vi "zmq REQ dup.vi"() -> ()   [LabVIEW 2015]
uses:
  <vilib>/addons/zeromq/poll_type.ctl
  <vilib>/addons/zeromq/socket_type.ctl
  <vilib>/addons/zeromq/zmq_context.lvclass
  <vilib>/addons/zeromq/zeromq.lvlib
  <vilib>/addons/zeromq/zmq_socket.lvclass
panel:
  in  "Connection Type":enum16{"connect", "bind"}(ring)
  in  "Poll":bool
  out "timed out?":bool
  out "nevents":i32
  out "polled events":T1[](array[typedef])
  in  "poll type":T1=enum."In/Out"
  in  "receive":bool
  in  "Message":string="{\"msg_id\":\"555\",\"msg_type\":\"read\",\"msg_property\":\"vmon\",\"8-04\":\"XXX\"}"
  in  "SEND":bool
  out "HB":bool
  out "error out":errorcluster
  in  "stop":bool
  in  "ZMQ endpoint":string="tcp://127.0.0.1:5555"
  out "REPLY":string
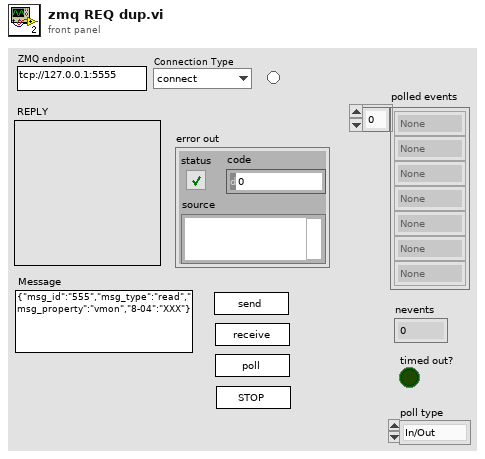
[diagram p1: front panel]
types:
  T1 = typedef "zeromq.lvlib/poll_type.ctl" = enum16{"None", "In", "Out", "In/Out"}
  T2 = typedef "zeromq.lvlib/socket_type.ctl" = enum8{"ZMQ_PAIR", "ZMQ_PUB", "ZMQ_SUB", "ZMQ_REQ", "ZMQ_REP", "ZMQ_DEALER", "ZMQ_ROUTER", "ZMQ_PULL", "ZMQ_PUSH", "ZMQ_XPUB", "ZMQ_XSUB"}
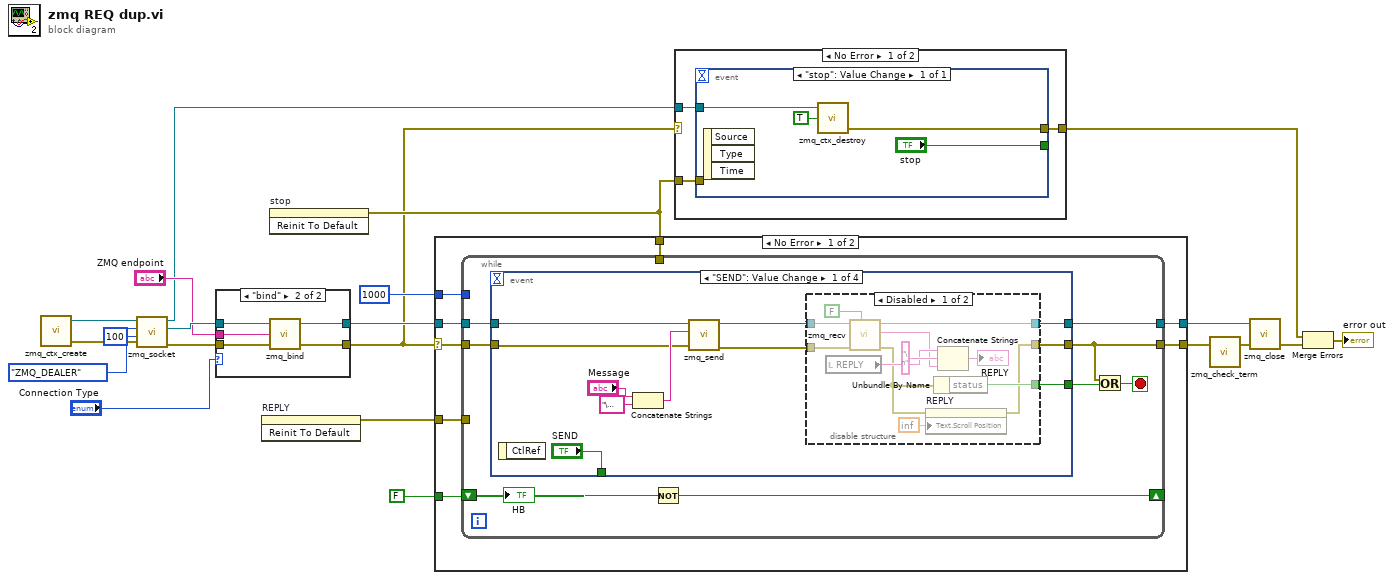
[diagram p0: block diagram]
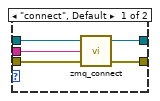
[diagram p2: hidden frame]
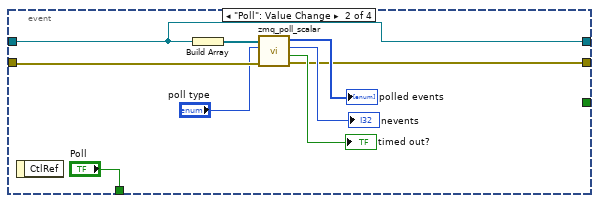
[diagram p4: hidden frame]
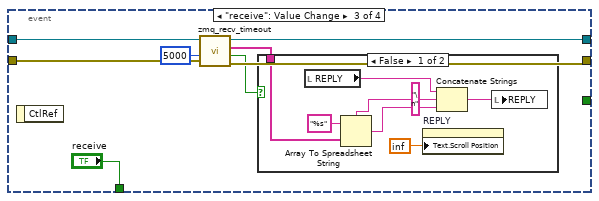
[diagram p5: hidden frame]
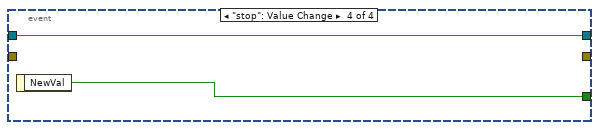
[diagram p7: hidden frame]
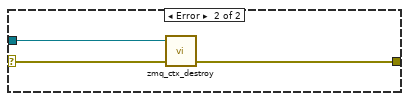
[diagram p9: hidden frame]
diagram:
  n1 = call <vilib>:"zmq_ctx_create.vi"() -> ("error out"=w14:errorcluster, "context out"=w12:refnum<class "zmq_context.lvclass">)  [unwired: 4 in]
  n2 = call <vilib>:"zmq_socket.vi"("error in"=w14, "linger (ms)"=100, "socket type"=socket_type."ZMQ_DEALER", "context in"=w12) -> ("error out"=w19:errorcluster, "socket out"=w20:refnum<class "zmq_socket.lvclass">, "context out"=w1:refnum<class "zmq_context.lvclass">)  [unwired: 1 in]
  n3 = case shown="\"bind\"" "Connection Type" {
    tunnel: w20 -> [w26 w31]
    tunnel: w19 -> [w25 w28]
    tunnel: [w24 w30] -> w18
    tunnel: "ZMQ endpoint" -> [w23 w27]
    tunnel: [w22 w29] -> w3
    frame "connect", Default {
      n4 = call <vilib>:"zmq_connect.vi"("error in"=w25, "endpoint"=w23, "socket in"=w26) -> ("error out"=w22:errorcluster, "socket out"=w24:refnum<class "zmq_socket.lvclass">)  [unwired: 1 in]
    }
    frame "bind" {
      n5 = call <vilib>:"zmq_bind.vi"("error in"=w28, "endpoint"=w27, "socket in"=w31) -> ("error out"=w29:errorcluster, "socket out"=w30:refnum<class "zmq_socket.lvclass">)  [unwired: 1 in]
    }
  }
  n6 = invoke on="REPLY" class="Str" method="Reinit To Default"() -> (error out=w13:errorcluster)  [unwired: 3 in, 2 out]
  n7 = invoke on="stop" class="Bool" method="Reinit To Default"() -> (error out=w5:errorcluster)  [unwired: 3 in, 2 out]
  n8 = case shown="No Error" w3 {
    selector: w3 -> [w32 w100]
    tunnel: w18 -> [w39 w99]
    tunnel: 1000 -> [w38 _]
    tunnel: [w37 w99] -> w16
    tunnel: w13 -> [w36 _]
    tunnel: [w35 w100] -> w11
    tunnel: FALSE ("stop") -> [w34 _]
    tunnel: w5 -> [w33 _]
    frame No Error {
      n9 = while {
        tunnel: w39 -> [w47]
        tunnel: w32 -> [w46]
        tunnel: w38 -> [_]
        tunnel: [w45] -> w37
        tunnel: [w40] -> w35
        tunnel: w36 -> [_]
        shift-right: [w43] -> _
        shift-left: w34 -> [w44]
        tunnel: w33 -> [_]
        stop <- w42 stop-if-true
        n10 = event shown="[0] \"SEND\": Value Change" {
          selector: _ -> [_ _ _ _]
          dyn-events: _ -> [_ _ _ _]
          timeout: _ -> [_ _ _ _]
          tunnel: [w57 _ _ w97] -> w41
          tunnel: w47 -> [w48 w75 w89 w98]
          tunnel: w46 -> [w49 w76 w88 _]
          tunnel: [w56 w75 w85 w98] -> w45
          tunnel: [w50 w74 w86 _] -> w40
          tunnel: ["SEND" "Poll" "receive" _] -> _
          event "SEND": Value Change {
            n11 = event-data() -> ()  [unwired: 1 in, 1 out]
            n12 = Concatenate Strings("Message", "\u0000" ("string")) -> (w51:string)
            n13 = call <vilib>:"zmq_send.vi"("error in"=w49, "data"=w51, "socket in"=w48) -> ("error out"=w55:errorcluster, "socket out"=w58:refnum<class "zmq_socket.lvclass">)  [unwired: 4 in]
            n14 = disable-structure shown="Disabled" {
              disable-tunnel: w58 -> [w70 w72]
              disable-tunnel: [w69 _] -> w57
              disable-tunnel: [w68 w72] -> w56
              disable-tunnel: w55 -> [w66 w71]
              disable-tunnel: [w59 w71] -> w50
              frame Disabled {
                n15 = local read "REPLY"() -> (w62:string)
                n16 = call <vilib>:"zmq_recv.vi"("no block? (F)"=FALSE, "error in"=w66, "socket in"=w70) -> ("error out"=w60:errorcluster, "data"=w61:string, "socket out"=w68:refnum<class "zmq_socket.lvclass">)  [unwired: 2 in, 2 out]
                n17 = property on="REPLY" class="Str"(error in=w60, "Text.Scroll Position"=inf) -> (error out=w59:errorcluster)  [unwired: 1 in, 1 out]
                n18 = Unbundle By Name(w60) -> ("status"=w69:bool)
                n19 = Concatenate Strings(w62, "\n" ("string"), w61) -> (→"REPLY":string)
              }
              frame Enabled {
              }
            }
          }
          event "Poll": Value Change {
            n20 = event-data() -> ()  [unwired: 1 in, 1 out]
            n21 = Build Array(w75) -> (w80:refnum<class "zmq_socket.lvclass">[])
            n22 = call <vilib>:"zmq_poll_scalar.vi"("error in"=w76, "poll type"="poll type", "sockets"=w80) -> ("error out"=w74:errorcluster, "timed out?"=→"timed out?":bool, "nevents"=→"nevents":i32, "polled events"=→"polled events":T1[])  [unwired: 1 in]
          }
          event "receive": Value Change {
            n23 = event-data() -> ()  [unwired: 1 in, 1 out]
            n24 = call <vilib>:"zmq_recv_timeout.vi"("error in"=w88, "timeout (ms)"=u32 5000, "socket in"=w89) -> ("error out"=w86:errorcluster, "timeout?"=w83:bool, "parts"=w84:string[], "socket out"=w85:refnum<class "zmq_socket.lvclass">)  [unwired: 1 in]
            n25 = case shown="False" w83 {
              tunnel: w84 -> [w92 _]
              frame False {
                w93 = "\n" ("string")
                n26 = local read "REPLY"() -> (w95:string)
                n27 = Array To Spreadsheet String(delimiter (Tab)=w93, array=w92, 3:"%s" ("format string")) -> (spreadsheet string=w91:string)
                n28 = property on="REPLY" class="Str"("Text.Scroll Position"=inf) -> ()  [unwired: 2 in, 2 out]
                n29 = Concatenate Strings(w95, w93, w91) -> (w96:string)
                n30 = local write "REPLY"(w96) -> ()
              }
              frame True {
              }
            }
          }
          event "stop": Value Change {
            n31 = event-data() -> ("NewVal"=w97:bool)  [unwired: 1 in]
          }
        }
        n32 = Not(x=w44) -> (.not. x?=w43:bool)
        n33 = Or(x=w40, y=w41) -> (x .or. y?=w42:bool)
        "HB" <- w44
      }
    }
    frame Error {
    }
  }
  n34 = case shown="No Error" w3 {
    selector: w3 -> [_ w109]
    tunnel: w1 -> [w103 w110]
    tunnel: [w102 w108] -> w8
    tunnel: w5 -> [w101 _]
    frame No Error {
      n35 = event shown="[0] \"stop\": Value Change" {
        selector: _ -> [_]
        dyn-events: _ -> [_]
        timeout: _ -> [_]
        tunnel: w103 -> [w107]
        tunnel: ["stop"] -> _
        tunnel: [w105] -> w102
        tunnel: w101 -> [_]
        event "stop": Value Change {
          n36 = event-data() -> ()  [unwired: 1 in, 3 out]
          n37 = call <vilib>:"zmq_ctx_destroy.vi"("reap? (F)"=TRUE, "context in"=w107) -> ("error out"=w105:errorcluster)  [unwired: 3 in]
        }
      }
    }
    frame Error {
      n38 = call <vilib>:"zmq_ctx_destroy.vi"("error in"=w109, "context in"=w110) -> ("error out"=w108:errorcluster)  [unwired: 3 in]
    }
  }
  n39 = call <vilib>:"zmq_check_term.vi"("error in"=w11) -> ("error out"=w10:errorcluster)  [unwired: 1 in, 1 out]
  n40 = call <vilib>:"zmq_close.vi"("error in"=w10, "socket"=w16) -> ("error out"=w9:errorcluster)  [unwired: 3 in]
  n41 = Merge Errors(w8, w9) -> (→"error out":errorcluster)
